vi "Queue FIFO（U32）.vi"(8 "error in (no error)":errorcluster caption="错误输入（无错误）", 9 "模式":enum16{"初始化", "加入元素", "当前队列", "释放"}(ring)=enum."加入元素", 10 "length":i32=100 caption="采样长度", 11 "输入":u32 caption="输入数据点") -> (0 "error out":errorcluster caption="错误输出", 1 "当前长度":i32, 2 "当前队列":u32[](array[numeric]), 3 "除去元素":u32)   [LabVIEW 2012, in "Queue FIFO.lvlib"]
uses:
  Queue FIFO.lvlib
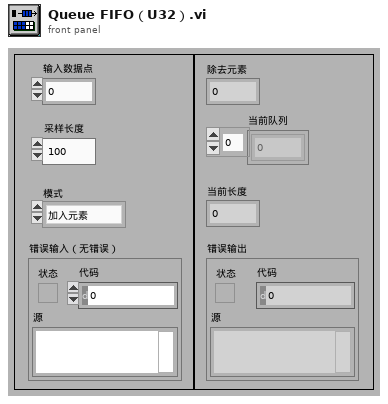
[diagram p1: front panel]
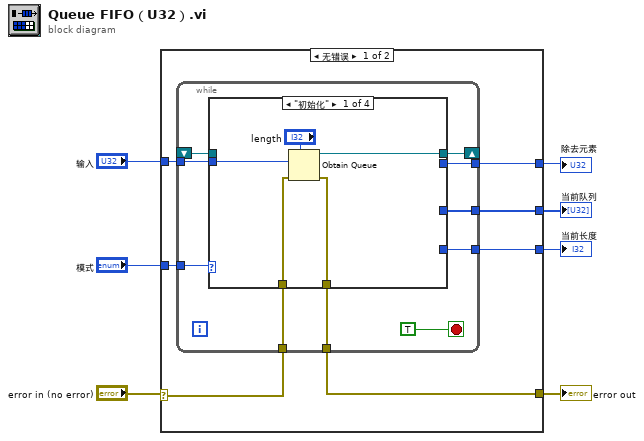
[diagram p0: block diagram]
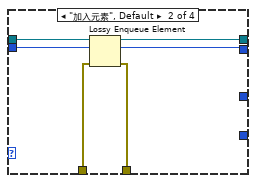
[diagram p2: hidden frame]
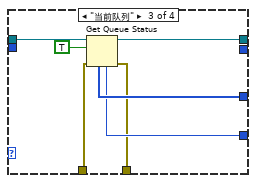
[diagram p3: hidden frame]
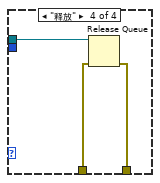
[diagram p4: hidden frame]
diagram:
  n1 = case shown="无错误" "error in (no error)" {
    selector: "error in (no error)" -> [w13 w46]
    tunnel: "模式" -> [w14 _]
    tunnel: [w12 w46] -> w5
    tunnel: "输入" -> [w11 _]
    tunnel: [w10 _] -> w3
    tunnel: [w9 _] -> w2
    tunnel: [w8 _] -> w1
    frame No Error {
      n2 = while {
        tunnel: w14 -> [w23]
        shift-right: [w20] -> _
        shift-left: _ -> [w19]
        tunnel: w13 -> [w22]
        tunnel: [w21] -> w12
        tunnel: w11 -> [w18]
        tunnel: [w17] -> w10
        tunnel: [w16] -> w9
        tunnel: [w15] -> w8
        stop <- TRUE stop-if-true
        n3 = case shown="\"初始化\"" w23 {
          tunnel: w22 -> [w29 w33 w38 w44]
          tunnel: [w28 w32 w37 w43] -> w21
          tunnel: [w27 w34 w41 _] -> w20
          tunnel: w19 -> [_ w35 w42 w45]
          tunnel: w18 -> [w25 w31 _ _]
          tunnel: [_ _ w40 _] -> w17
          tunnel: [_ _ w39 _] -> w16
          tunnel: [_ w30 _ _] -> w15
          frame "初始化" {
            n4 = Obtain Queue(max queue size (-1, unlimited)="length", element data type=w25, error in (no error)=w29) -> (queue out=w27:refnum<queue>, error out=w28:errorcluster)  [unwired: 2 in, 1 out]
          }
          frame "加入元素", Default {
            n5 = Lossy Enqueue Element(queue=w35, element=w31, error in (no error)=w33) -> (queue out=w34:refnum<queue>, overflow element=w30:u32, error out=w32:errorcluster)  [unwired: 1 out]
          }
          frame "当前队列" {
            n6 = Get Queue Status(queue=w42, return elements? (F)=TRUE ("返回元素？(F)"), error in (no error)=w38) -> (queue out=w41:refnum<queue>, error out=w37:errorcluster, # elements in queue=w39:i32, elements=w40:u32[])  [unwired: 4 out]
          }
          frame "释放" {
            n7 = Release Queue(queue=w45, error in (no error)=w44) -> (error out=w43:errorcluster)  [unwired: 1 in, 2 out]
          }
        }
      }
    }
    frame Error {
    }
  }
  "当前队列" <- w3
  "当前长度" <- w2
  "error out" <- w5
  "除去元素" <- w1
